vi "Active GU Arrange List Menu.vi"(8 "error in":errorcluster, 9 "Point":T1, 10 "MenuRef":refnum<k9>, 11 "CtlRef":refnum<vi>) -> (0 "error out":errorcluster)   [LabVIEW 2020, in "GUCalibration2.lvlib"]
uses:
  GUCalibration2.lvlib
  <vilib>/Utility/miscctls.llb/LVPositionTypeDef.ctl
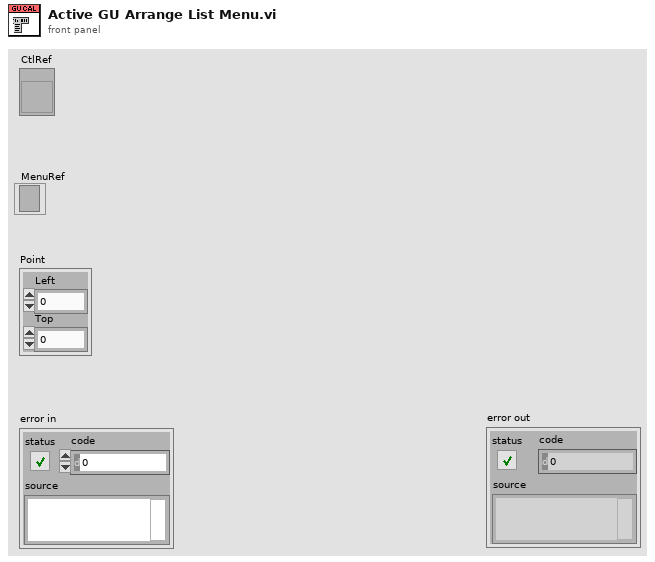
[diagram p1: front panel]
types:
  T1 = typedef "LVPositionTypeDef.ctl" = cluster{"Left":i32, "Top":i32}
  T2 = typedef "LVRowAndColumnTypeDef.ctl" = cluster{"Row":i32, "Column":i32}
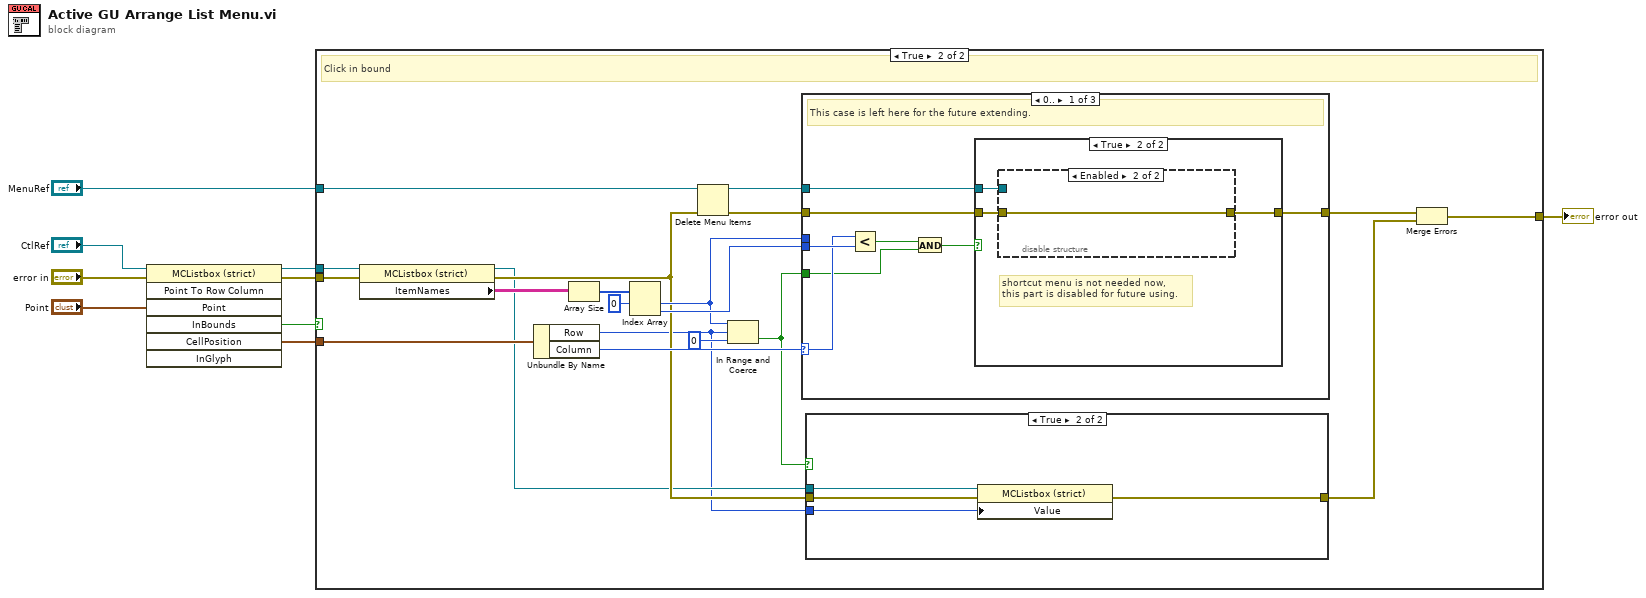
[diagram p0: block diagram]
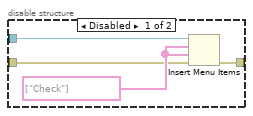
[diagram p5: hidden frame]
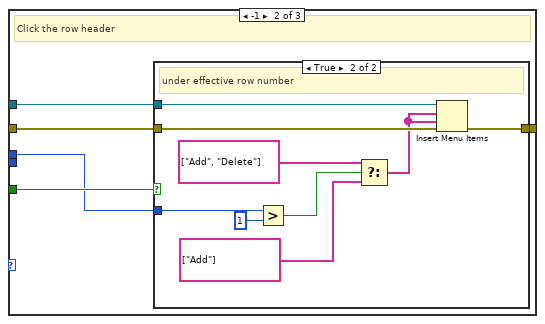
[diagram p6: hidden frame]
diagram:
  n1 = invoke class="MCListbox (strict)" method="Point To Row Column"(reference="CtlRef", error in="error in", "Point"="Point") -> (reference out=w7:refnum<vi>, error out=w6:errorcluster, "InBounds"=w1:bool, "CellPosition"=w5:T2)  [unwired: 4 in, 3 out]
  n2 = case shown="True" w1 {
    tunnel: w7 -> [_ w30]
    tunnel: w6 -> [w10 w29]
    tunnel: w5 -> [_ w26]
    tunnel: "MenuRef" -> [_ w25]
    tunnel: [w10 w11] -> w2
    frame False {
    }
    frame True {
      # "Click in bound"
      n3 = property class="MCListbox (strict)"(reference=w30, error in=w29) -> (reference out=w15:refnum<vi>, error out=w16:errorcluster, "ItemNames"=w28:string[][])
      n4 = Unbundle By Name(w26) -> ("Row"=w14:i32, "Column"=w22:i32)
      n5 = Array Size(array=w28) -> (size(s)=w27:i32[])
      n6 = Index Array(array=w27, index #1=0 ("index")) -> (element #1=w18:i32, element #2=w20:i32)  [unwired: 1 in]
      n7 = Delete Menu Items(6:w16, 9:w25) -> (0:w23:errorcluster, 3:w24:refnum<k9>)  [unwired: 2 in]
      n8 = In Range and Coerce(upper limit=w18, x=w14, lower limit=0) -> (In Range?=w17:bool)  [unwired: 1 out]
      n9 = case shown="0.." w22 {
        selector: w22 -> [w37 _ _]
        tunnel: w24 -> [w39 w57 _]
        tunnel: w23 -> [w42 w56 w68]
        tunnel: [w38 w55 w68] -> w13
        tunnel: w20 -> [w43 _ _]
        tunnel: w17 -> [w36 w54 _]
        tunnel: w18 -> [_ w53 _]
        frame 0.. {
          # "This case is left here for the future extending."
          n10 = Less?(x=w37, y=w43) -> (x < y?=w41:bool)
          n11 = And(x=w41, y=w36) -> (x .and. y?=w40:bool)
          n12 = case shown="True" w40 {
            tunnel: w42 -> [w44 w45]
            tunnel: w39 -> [_ w47]
            tunnel: [w44 w46] -> w38
            frame False {
            }
            frame True {
              # "shortcut menu is not needed now,\nthis part is disabled for future using."
              n13 = disable-structure shown="Enabled" {
                disable-tunnel: w47 -> [w51 _]
                disable-tunnel: [w49 w52] -> w46
                disable-tunnel: w45 -> [w48 w52]
                frame Disabled {
                  w50 = string[] ["Check"] ("item names")
                  n14 = Insert Menu Items(6:w48, 7:w50, 8:w50, 9:w51) -> (0:w49:errorcluster)  [unwired: 2 in, 2 out]
                }
                frame Enabled {
                }
              }
            }
          }
        }
        frame -1 {
          # "Click the row header"
          n15 = case shown="True" w54 {
            tunnel: w57 -> [_ w67]
            tunnel: w56 -> [w58 w66]
            tunnel: [w58 w65] -> w55
            tunnel: w53 -> [_ w59]
            frame False {
            }
            frame True {
              # "under effective row number"
              n16 = Greater?(x=w59, y=1) -> (0:w63:bool)
              n17 = Select(t=string[] ["Add", "Delete"] ("item names"), s=w63, f=string[] ["Add"] ("item names")) -> (s? t:f=w61:string[])
              n18 = Insert Menu Items(6:w66, 7:w61, 8:w61, 9:w67) -> (0:w65:errorcluster)  [unwired: 2 in, 2 out]
            }
          }
        }
        frame -2, Default {
        }
      }
      n19 = case shown="True" w17 {
        tunnel: w16 -> [w31 w35]
        tunnel: w15 -> [_ w34]
        tunnel: w14 -> [_ w33]
        tunnel: [w31 w32] -> w12
        frame False {
        }
        frame True {
          n20 = property class="MCListbox (strict)"(reference=w34, error in=w35, "Value"=w33) -> (error out=w32:errorcluster)  [unwired: 1 out]
        }
      }
      n21 = Merge Errors(w13, w12) -> (w11:errorcluster)
    }
  }
  "error out" <- w2
